vi "Set_Calibration_Settings.vi"(8 "Status/Errors in":refnum<vi>, 9 "Control Parameters [] in":T1[](array[typedef]) {"Aux Byte Value" format="%02x"; "Max Real Value" format="%#_6e"; "Min Real Value" format="%#_6e"; "dReal/dByte" format="%#_6e"; "Byte Value" format="%02x"; "Identifier" format="%02x"}, 10 "Main parameters in":T3={"Mode"={"Mode"=enum."Dialog", "Expert?"=FALSE, "Dialog?"=FALSE}, "Stop loop"={"Settings changed?"=FALSE, "Stop?"=refnum}, "Send message"={"Send mode"=enum."Get parameters", "Set parameter list"=0, "Get parameter list"=0, "Reset device"=0, "Length set settings message"=0, "Reset buttons?"=FALSE, "Reset Master?"=enum."General"}, "Write settings"={"Options"=enum."File 1"}, "Settings state"={"MAS locked?"=refnum, "SLV locked?"=refnum}, "Button refs"={"Stop program"=refnum, "Save settings"=refnum, "DAQ mode"=refnum, "Reset settings"=refnum, "Apply settings"=refnum, "Reset MAS"=refnum, "Reset SLV"=refnum, "Local DBase?"=refnum, "Last value DBase"=FALSE, "Database"=refnum, "Calibration"=refnum, "Save settings 2"=refnum}, "Update screen"={"Detector number"=0, "Hardware"=enum."None"}, "Files"={"Path config file"=path "", "Path def. ini file"=path "", "Path ini file 1"=path "", "Path ini file 2"=path "", "Path RBF file"=path ""}, "DB connection"={"connection reference"=refnum, "Connected?"=refnum, "ODBC Name"=""}, "Status_id"=refnum, "Time difference"=refnum, "Satellites"=refnum, "Alignment parameters"=refnum, "Page Statistics 2"=refnum, "Database"=refnum, "Page Statistics"=refnum} {"Update screen"."Detector number" format="%#.0f"; "Send message"."Reset device" format="%x"; "Send message"."Get parameter list" format="%x"; "Send message"."Set parameter list" format="%x"}) -> (0 "Status/Errors out":refnum<vi>, 1 "Control Parameters [] out":T1[](array[typedef]) {"Aux Byte Value" format="%02x"; "Max Real Value" format="%#_6e"; "Min Real Value" format="%#_6e"; "dReal/dByte" format="%#_6e"; "Byte Value" format="%02x"; "Identifier" format="%02x"}, 2 "Main parameters out":T3={"Mode"={"Mode"=enum."Dialog", "Expert?"=FALSE, "Dialog?"=FALSE}, "Stop loop"={"Settings changed?"=FALSE, "Stop?"=refnum}, "Send message"={"Send mode"=enum."Get parameters", "Set parameter list"=0, "Get parameter list"=0, "Reset device"=0, "Length set settings message"=0, "Reset buttons?"=FALSE, "Reset Master?"=enum."General"}, "Write settings"={"Options"=enum."File 1"}, "Settings state"={"MAS locked?"=refnum, "SLV locked?"=refnum}, "Button refs"={"Stop program"=refnum, "Save settings"=refnum, "DAQ mode"=refnum, "Reset settings"=refnum, "Apply settings"=refnum, "Reset MAS"=refnum, "Reset SLV"=refnum, "Local DBase?"=refnum, "Last value DBase"=FALSE, "Database"=refnum, "Calibration"=refnum, "Save settings 2"=refnum}, "Update screen"={"Detector number"=0, "Hardware"=enum."None"}, "Files"={"Path config file"=path "", "Path def. ini file"=path "", "Path ini file 1"=path "", "Path ini file 2"=path "", "Path RBF file"=path ""}, "DB connection"={"connection reference"=refnum, "Connected?"=refnum, "ODBC Name"=""}, "Status_id"=refnum, "Time difference"=refnum, "Satellites"=refnum, "Alignment parameters"=refnum, "Page Statistics 2"=refnum, "Database"=refnum, "Page Statistics"=refnum} {"Update screen"."Detector number" format="%#.0f"; "Send message"."Reset device" format="%x"; "Send message"."Get parameter list" format="%x"; "Send message"."Set parameter list" format="%x"})   [LabVIEW 2010]
uses:
  Controls/Main_Parameters.ctl
  Controls/Mode.ctl
  Controls/Stop_Loop.ctl
  Controls/Send_Message.ctl
  Controls/Send_Message_Mode.ctl
  Controls/Master.ctl
  Controls/Write_Settings.ctl
  Controls/Write_Settings_Options.ctl
  Controls/Settings_State.ctl
  Controls/Button_Refs.ctl
  Controls/Update_Screen.ctl
  Controls/Files.ctl
  Controls/DB_Connection.ctl
  database/Connection.llb/Conn ObjectReference.ctl
  Controls/Control_Parameters.ctl
  Controls/Get_Set_Calibration_Options.ctl
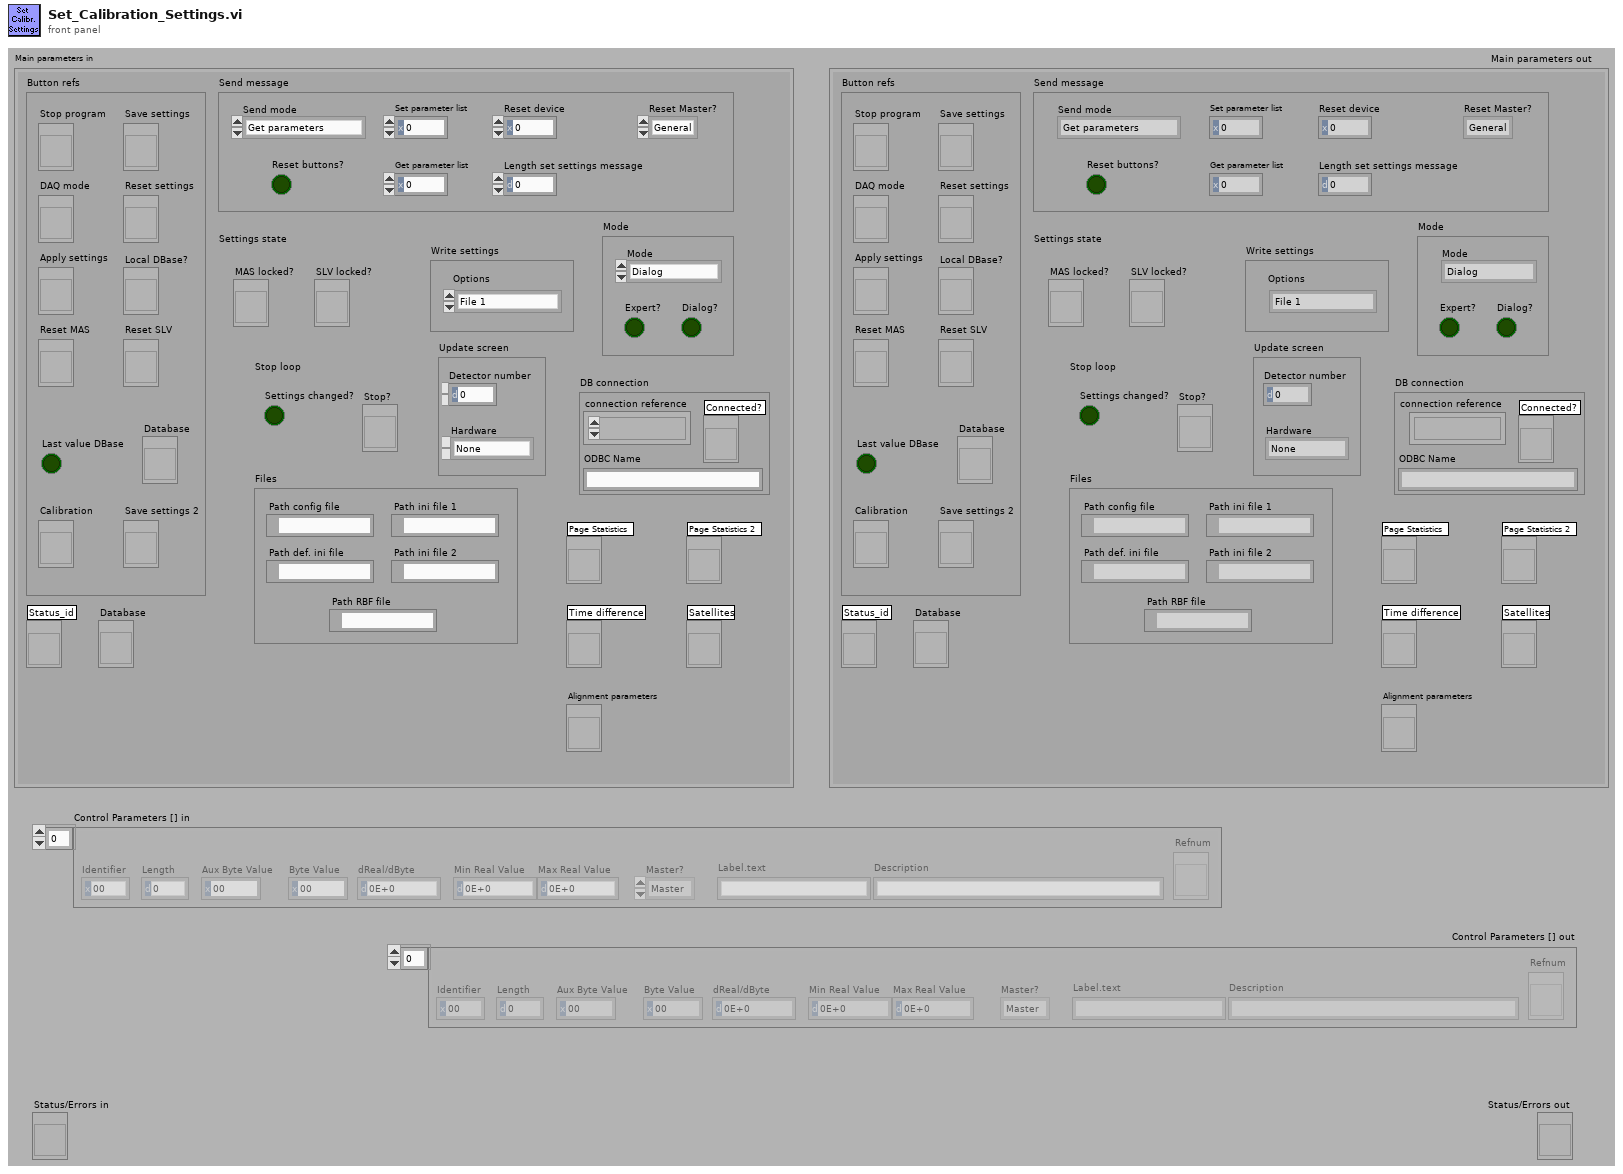
[diagram p1: front panel]
types:
  T1 = typedef "Control_Parameters.ctl" = cluster{"Identifier":u8, "Length":u16, "Byte Value":u32, "dReal/dByte":dbl, "Min Real Value":dbl, "Max Real Value":dbl, "Master?":T2, "Label.text":string, "Description":string, "Refnum":refnum<vi>, "Aux Byte Value":u32}
  T2 = typedef "Master.ctl" = enum16{"Master", "Slave", "General"}
  T3 = typedef "Main_Parameters.ctl" = cluster{"Mode":T4, "Stop loop":T5, "Send message":T6, "Write settings":T8, "Settings state":T10, "Button refs":T11, "Update screen":T12, "Files":T13, "DB connection":T14, "Status_id":refnum<vi>, "Time difference":refnum<vi>, "Satellites":refnum<vi>, "Alignment parameters":refnum<vi>, "Page Statistics 2":refnum<vi>, "Database":refnum<vi>, "Page Statistics":refnum<vi>}
  T4 = typedef "Mode.ctl" = cluster{"Mode":enum8{"Stop", "Dialog", "Hisparc II", "Hisparc II DAQ", "Alignment"}, "Expert?":bool, "Dialog?":bool}
  T5 = typedef "Stop_Loop.ctl" = cluster{"Settings changed?":bool, "Stop?":refnum<vi>}
  T6 = typedef "Send_Message.ctl" = cluster{"Send mode":T7, "Set parameter list":u8, "Get parameter list":u8, "Reset device":u8, "Length set settings message":i32, "Reset buttons?":bool, "Reset Master?":T2}
  T7 = typedef "Send_Message_Mode.ctl" = enum16{"Get parameters", "Set parameters", "From front panel", "From parameters", "Reset device", "Alignment"}
  T8 = typedef "Write_Settings.ctl" = cluster{"Options":T9}
  T9 = typedef "Write_Settings_Options.ctl" = enum16{"File 1", "File 2", "Alignment", "Reset"}
  T10 = typedef "Settings_State.ctl" = cluster{"MAS locked?":refnum<vi>, "SLV locked?":refnum<vi>}
  T11 = typedef "Button_Refs.ctl" = cluster{"Stop program":refnum<vi>, "Save settings":refnum<vi>, "DAQ mode":refnum<vi>, "Reset settings":refnum<vi>, "Apply settings":refnum<vi>, "Reset MAS":refnum<vi>, "Reset SLV":refnum<vi>, "Local DBase?":refnum<vi>, "Last value DBase":bool, "Database":refnum<vi>, "Calibration":refnum<vi>, "Save settings 2":refnum<vi>}
  T12 = typedef "Update_Screen.ctl" = cluster{"Detector number":u16, "Hardware":enum8{"None", "HiSPARC I", "HiSPARC II", "HiSPARC III", "Unknown"}}
  T13 = typedef "Files.ctl" = cluster{"Path config file":path, "Path def. ini file":path, "Path ini file 1":path, "Path ini file 2":path, "Path RBF file":path}
  T14 = typedef "DB_Connection.ctl" = cluster{"connection reference":T15, "Connected?":refnum<vi>, "ODBC Name":string}
  T15 = typedef "Conn ObjectReference.ctl" = refnum<k1>
  T16 = typedef "Get_Set_Calibration_Options.ctl" = enum16{"Get", "Set", "Set MAS", "Set SLV"}
  T17 = typedef "Calibration_Parameters.ctl" = cluster{"New settings MAS?":bool, "New settings SLV?":bool, "Alignment step MAS":i32, "Alignment step SLV":i32, "MAS Ch. 1":cluster{"Offset adjust pos.":u8, "Offset adjust neg.":u8, "Gain adjust pos.":u8, "Gain adjust neg.":u8, "Count pos.":dbl, "Count neg.":dbl}, "MAS Ch. 2":cluster{"Offset adjust pos.":u8, "Offset adjust neg.":u8, "Gain adjust pos.":u8, "Gain adjust neg.":u8, "Count pos.":dbl, "Count neg.":dbl}, "SLV Ch. 1":cluster{"Offset adjust pos.":u8, "Offset adjust neg.":u8, "Gain adjust pos.":u8, "Gain adjust neg.":u8, "Count pos.":dbl, "Count neg.":dbl}, "SLV Ch. 2":cluster{"Offset adjust pos.":u8, "Offset adjust neg.":u8, "Gain adjust pos.":u8, "Gain adjust neg.":u8, "Count pos.":dbl, "Count neg.":dbl}, "Comm. offset MAS":u8, "Full scale MAS":u8, "Comm. offset SLV":u8, "Full scale SLV":u8, "Trigger condition":u8, "Pre coinc. time":u16, "Coinc. time":u16, "Post coinc. time":u16, "Hardware":enum8{"None", "HiSPARC I", "HiSPARC II", "HiSPARC III", "Unknown"}}
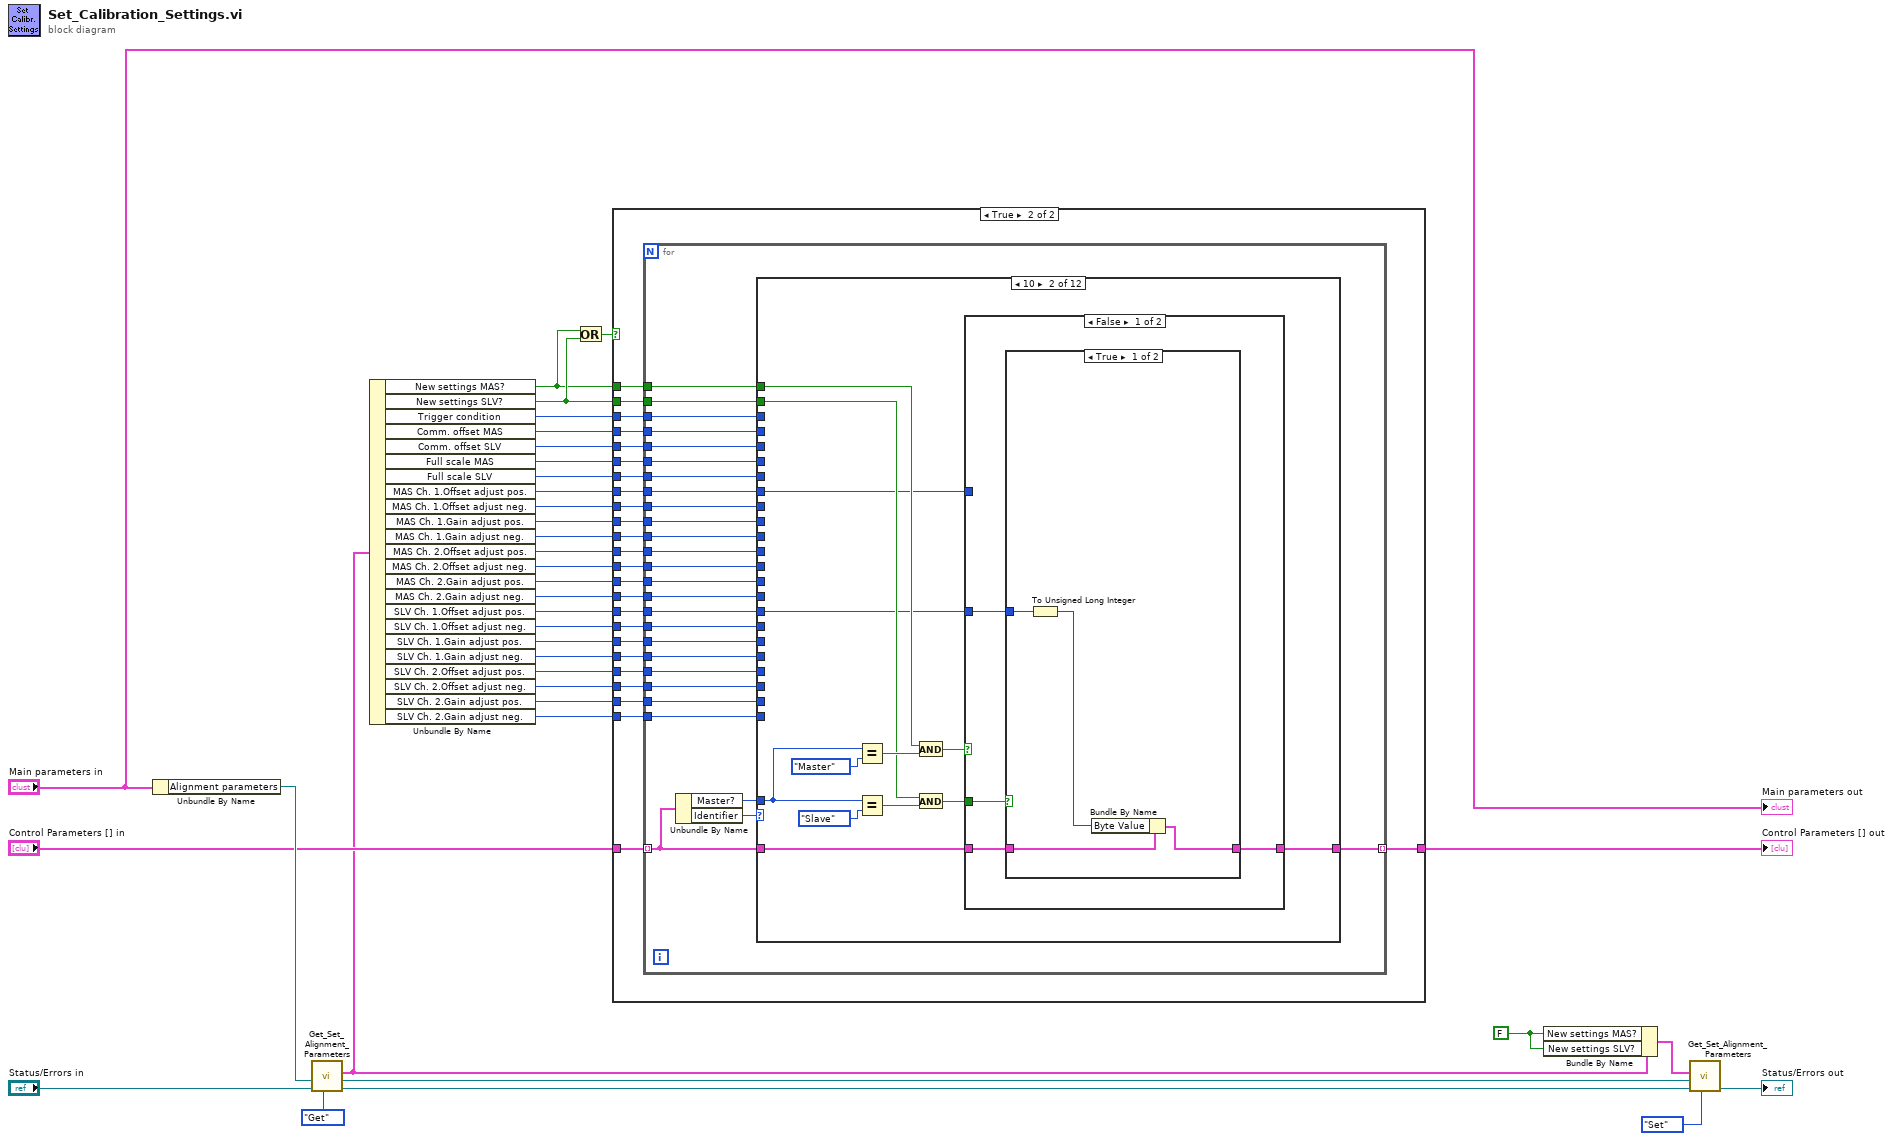
[diagram p0: block diagram]
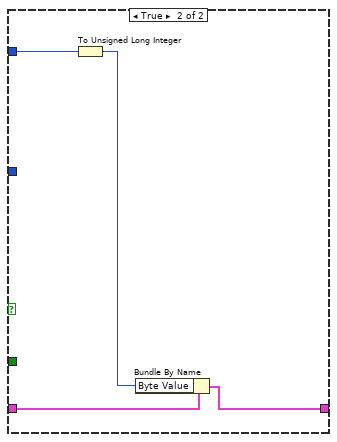
[diagram p5: hidden frame]
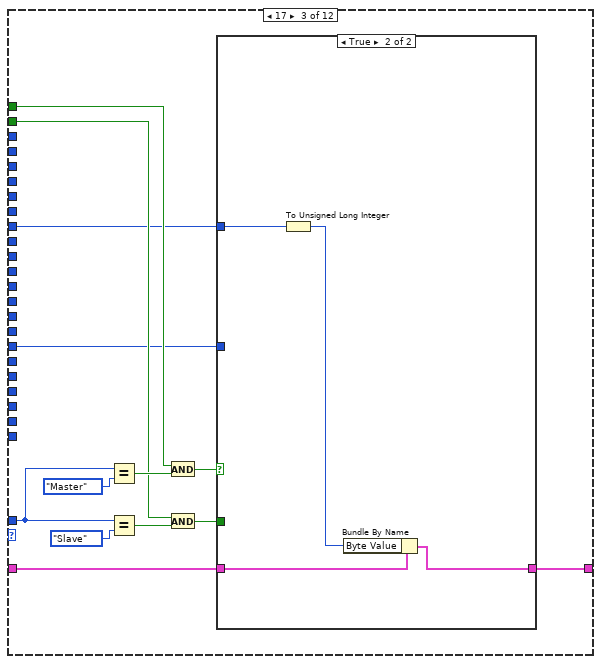
[diagram p6: hidden frame]
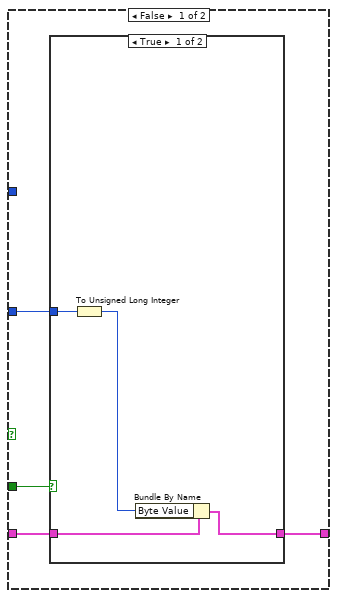
[diagram p7: hidden frame]
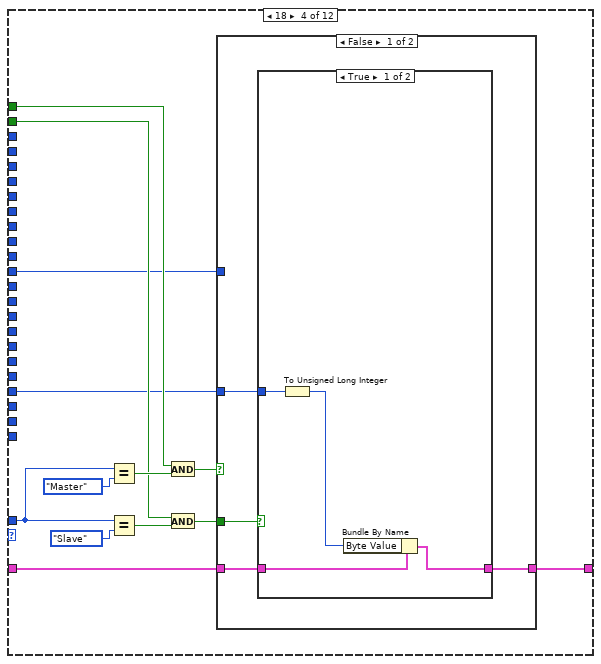
[diagram p9: hidden frame]
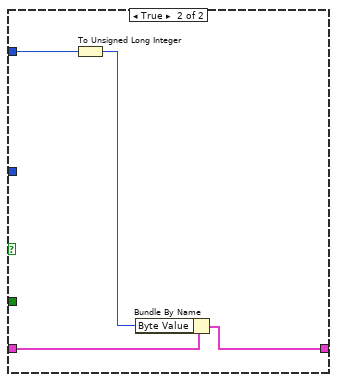
[diagram p11: hidden frame]
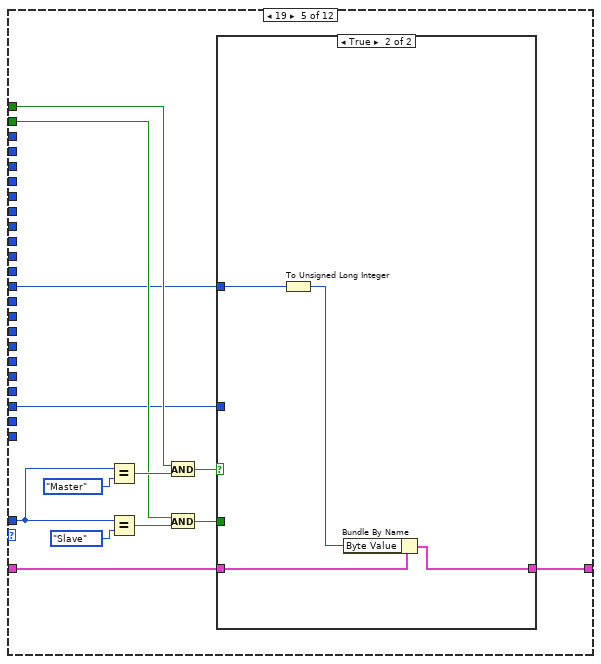
[diagram p12: hidden frame]
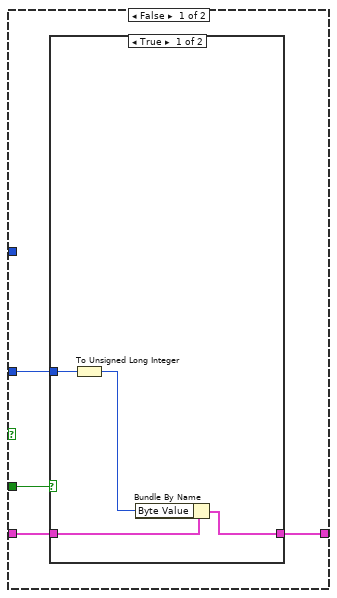
[diagram p13: hidden frame]
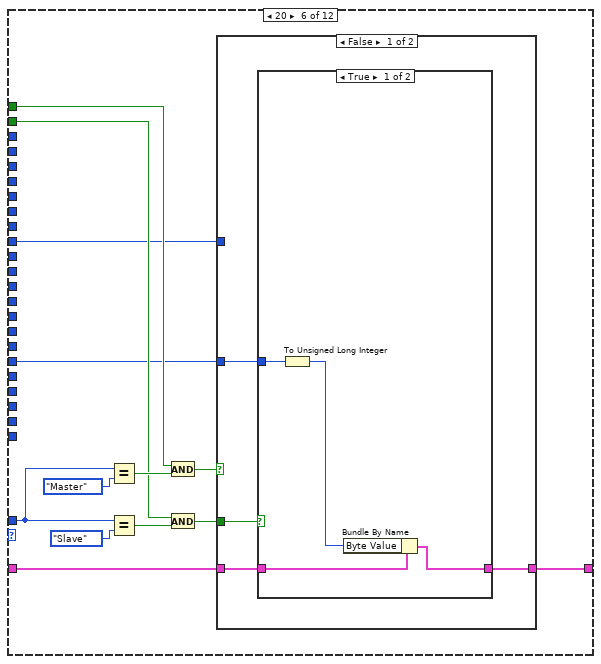
[diagram p15: hidden frame]
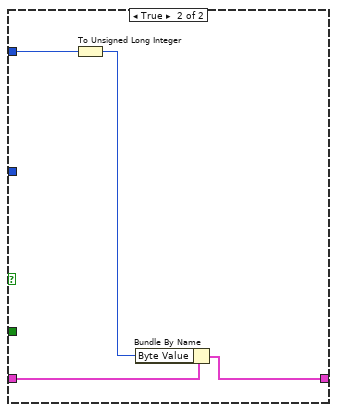
[diagram p17: hidden frame]
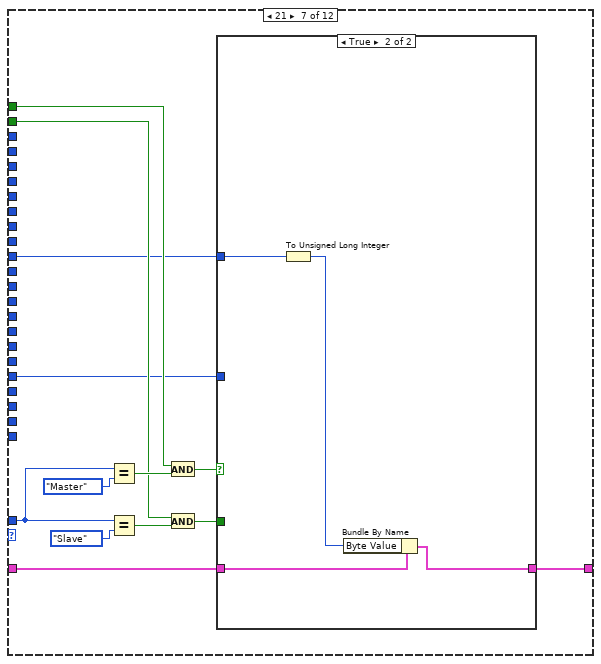
[diagram p18: hidden frame]
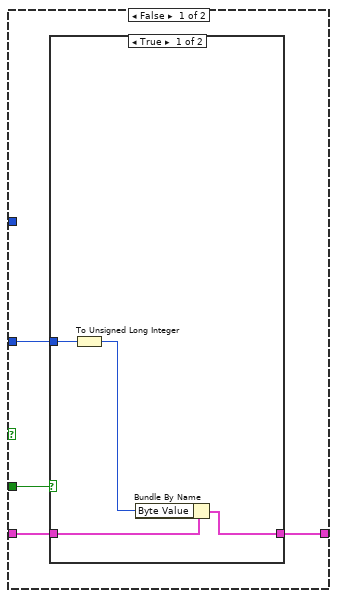
[diagram p19: hidden frame]
diagram:
  w6 = FALSE ("New settings MAS?")
  n1 = Unbundle By Name("Main parameters in") -> ("Alignment parameters"=w35:refnum<vi>)
  n2 = call "Get_Set_Alignment_Parameters.vi"("Get/Set"=Get_Set_Calibration_Options."Get", "Status/Errors in"="Status/Errors in", "Alignment parameters in"=w35) -> ("Status/Errors out"=w11:refnum<vi>, "Alignment parameters out"=w7:refnum<vi>, "Value out"=w9:T17)  [unwired: 2 in, 4 out]
  n3 = Unbundle By Name(w9) -> ("New settings MAS?"=w3:bool, "New settings SLV?"=w4:bool, "Trigger condition"=w31:u8, "Comm. offset MAS"=w30:u8, "Comm. offset SLV"=w2:u8, "Full scale MAS"=w29:u8, "Full scale SLV"=w1:u8, "MAS Ch. 1.Offset adjust pos."=w28:u8, "MAS Ch. 1.Offset adjust neg."=w27:u8, "MAS Ch. 1.Gain adjust pos."=w26:u8, "MAS Ch. 1.Gain adjust neg."=w25:u8, "MAS Ch. 2.Offset adjust pos."=w24:u8, "MAS Ch. 2.Offset adjust neg."=w23:u8, "MAS Ch. 2.Gain adjust pos."=w22:u8, "MAS Ch. 2.Gain adjust neg."=w21:u8, "SLV Ch. 1.Offset adjust pos."=w20:u8, "SLV Ch. 1.Offset adjust neg."=w19:u8, "SLV Ch. 1.Gain adjust pos."=w18:u8, "SLV Ch. 1.Gain adjust neg."=w17:u8, "SLV Ch. 2.Offset adjust pos."=w16:u8, "SLV Ch. 2.Offset adjust neg."=w15:u8, "SLV Ch. 2.Gain adjust pos."=w14:u8, "SLV Ch. 2.Gain adjust neg."=w13:u8)
  n4 = Or(x=w3, y=w4) -> (x .or. y?=w5:bool)
  n5 = case shown="True" w5 {
    tunnel: "Control Parameters [] in" -> [w38 w63]
    tunnel: w3 -> [_ w62]
    tunnel: w4 -> [_ w61]
    tunnel: [w38 w60] -> w33
    tunnel: w31 -> [_ w59]
    tunnel: w30 -> [_ w58]
    tunnel: w29 -> [_ w57]
    tunnel: w28 -> [_ w56]
    tunnel: w27 -> [_ w55]
    tunnel: w26 -> [_ w54]
    tunnel: w25 -> [_ w53]
    tunnel: w24 -> [_ w52]
    tunnel: w23 -> [_ w51]
    tunnel: w22 -> [_ w50]
    tunnel: w21 -> [_ w49]
    tunnel: w20 -> [_ w48]
    tunnel: w19 -> [_ w47]
    tunnel: w18 -> [_ w46]
    tunnel: w17 -> [_ w45]
    tunnel: w16 -> [_ w44]
    tunnel: w15 -> [_ w43]
    tunnel: w14 -> [_ w42]
    tunnel: w13 -> [_ w41]
    tunnel: w2 -> [_ w40]
    tunnel: w1 -> [_ w39]
    frame False {
    }
    frame True {
      n6 = for {
        tunnel: w63 -> [w67] mode=indexing
        tunnel: w62 -> [w89]
        tunnel: w61 -> [w88]
        tunnel: [w68] -> w60 mode=indexing
        tunnel: w59 -> [w87]
        tunnel: w58 -> [w86]
        tunnel: w57 -> [w85]
        tunnel: w56 -> [w84]
        tunnel: w55 -> [w83]
        tunnel: w54 -> [w82]
        tunnel: w53 -> [w81]
        tunnel: w52 -> [w80]
        tunnel: w51 -> [w79]
        tunnel: w50 -> [w78]
        tunnel: w49 -> [w77]
        tunnel: w48 -> [w76]
        tunnel: w47 -> [w75]
        tunnel: w46 -> [w74]
        tunnel: w45 -> [w73]
        tunnel: w44 -> [w72]
        tunnel: w43 -> [w71]
        tunnel: w42 -> [w70]
        tunnel: w41 -> [w69]
        tunnel: w40 -> [w65]
        tunnel: w39 -> [w64]
        n7 = Unbundle By Name(w67) -> ("Master?"=w66:T2, "Identifier"=w90:u8)
        n8 = case shown="10" w90 {
          tunnel: w89 -> [_ w97 w123 w149 w175 w201 w227 w253 w279 w305 w331 _]
          tunnel: w88 -> [_ w96 w122 w148 w174 w200 w226 w252 w278 w304 w330 _]
          tunnel: w87 -> [_ _ _ _ _ _ _ _ _ _ _ w352]
          tunnel: w86 -> [_ _ _ _ _ _ _ _ _ w300 _ _]
          tunnel: w85 -> [_ _ _ _ _ _ _ _ _ _ w327 _]
          tunnel: w84 -> [_ w93 _ _ _ _ _ _ _ _ _ _]
          tunnel: w83 -> [_ _ w119 _ _ _ _ _ _ _ _ _]
          tunnel: w82 -> [_ _ _ _ _ w197 _ _ _ _ _ _]
          tunnel: w81 -> [_ _ _ _ _ _ w223 _ _ _ _ _]
          tunnel: w80 -> [_ _ _ w145 _ _ _ _ _ _ _ _]
          tunnel: w79 -> [_ _ _ _ w171 _ _ _ _ _ _ _]
          tunnel: w78 -> [_ _ _ _ _ _ _ w249 _ _ _ _]
          tunnel: w77 -> [_ _ _ _ _ _ _ _ w275 _ _ _]
          tunnel: w76 -> [_ w92 _ _ _ _ _ _ _ _ _ _]
          tunnel: w75 -> [_ _ w118 _ _ _ _ _ _ _ _ _]
          tunnel: w74 -> [_ _ _ _ _ w196 _ _ _ _ _ _]
          tunnel: w73 -> [_ _ _ _ _ _ w222 _ _ _ _ _]
          tunnel: w72 -> [_ _ _ w144 _ _ _ _ _ _ _ _]
          tunnel: w71 -> [_ _ _ _ w170 _ _ _ _ _ _ _]
          tunnel: w70 -> [_ _ _ _ _ _ _ w248 _ _ _ _]
          tunnel: w69 -> [_ _ _ _ _ _ _ _ w274 _ _ _]
          tunnel: [w91 w104 w130 w156 w182 w208 w234 w260 w286 w312 w338 w353] -> w68
          tunnel: w67 -> [w91 w103 w129 w155 w181 w207 w233 w259 w285 w311 w337 w354]
          tunnel: w66 -> [_ w98 w124 w150 w176 w202 w228 w254 w280 w306 w332 _]
          tunnel: w65 -> [_ _ _ _ _ _ _ _ _ w301 _ _]
          tunnel: w64 -> [_ _ _ _ _ _ _ _ _ _ w326 _]
          frame Default {
          }
          frame 16 {
            n9 = Equal?(x=w98, y=Master."Master") -> (x = y?=w99:bool)
            n10 = Equal?(x=w98, y=Master."Slave") -> (x = y?=w101:bool)
            n11 = And(x=w97, y=w99) -> (x .and. y?=w95:bool)
            n12 = And(x=w96, y=w101) -> (x .and. y?=w94:bool)
            n13 = case shown="False" w95 {
              tunnel: [w108 w115] -> w104
              tunnel: w103 -> [w107 w116]
              tunnel: w94 -> [w106 _]
              tunnel: w93 -> [_ w114]
              tunnel: w92 -> [w105 _]
              frame False {
                n14 = case shown="True" w106 {
                  tunnel: [w112 w113] -> w108
                  tunnel: w107 -> [w111 w113]
                  tunnel: w105 -> [w110 _]
                  frame True {
                    n15 = To Unsigned Long Integer(number=w110) -> (unsigned 32bit integer=w109:u32)
                    n16 = Bundle By Name(cluster=w111, "Byte Value"=w109) -> (w112:T1)
                  }
                  frame False, Default {
                  }
                }
              }
              frame True {
                n17 = To Unsigned Long Integer(number=w114) -> (unsigned 32bit integer=w117:u32)
                n18 = Bundle By Name(cluster=w116, "Byte Value"=w117) -> (w115:T1)
              }
            }
          }
          frame 17 {
            n19 = Equal?(x=w124, y=Master."Master") -> (x = y?=w125:bool)
            n20 = Equal?(x=w124, y=Master."Slave") -> (x = y?=w127:bool)
            n21 = And(x=w123, y=w125) -> (x .and. y?=w121:bool)
            n22 = And(x=w122, y=w127) -> (x .and. y?=w120:bool)
            n23 = case shown="True" w121 {
              tunnel: [w134 w141] -> w130
              tunnel: w129 -> [w133 w142]
              tunnel: w120 -> [w132 _]
              tunnel: w118 -> [w131 _]
              tunnel: w119 -> [_ w140]
              frame False {
                n24 = case shown="True" w132 {
                  tunnel: [w138 w139] -> w134
                  tunnel: w133 -> [w137 w139]
                  tunnel: w131 -> [w136 _]
                  frame True {
                    n25 = To Unsigned Long Integer(number=w136) -> (unsigned 32bit integer=w135:u32)
                    n26 = Bundle By Name(cluster=w137, "Byte Value"=w135) -> (w138:T1)
                  }
                  frame False, Default {
                  }
                }
              }
              frame True {
                n27 = To Unsigned Long Integer(number=w140) -> (unsigned 32bit integer=w143:u32)
                n28 = Bundle By Name(cluster=w142, "Byte Value"=w143) -> (w141:T1)
              }
            }
          }
          frame 18 {
            n29 = Equal?(x=w150, y=Master."Master") -> (x = y?=w151:bool)
            n30 = Equal?(x=w150, y=Master."Slave") -> (x = y?=w153:bool)
            n31 = And(x=w149, y=w151) -> (x .and. y?=w147:bool)
            n32 = And(x=w148, y=w153) -> (x .and. y?=w146:bool)
            n33 = case shown="False" w147 {
              tunnel: [w160 w167] -> w156
              tunnel: w155 -> [w159 w168]
              tunnel: w146 -> [w158 _]
              tunnel: w144 -> [w157 _]
              tunnel: w145 -> [_ w166]
              frame False {
                n34 = case shown="True" w158 {
                  tunnel: [w164 w165] -> w160
                  tunnel: w159 -> [w163 w165]
                  tunnel: w157 -> [w162 _]
                  frame True {
                    n35 = To Unsigned Long Integer(number=w162) -> (unsigned 32bit integer=w161:u32)
                    n36 = Bundle By Name(cluster=w163, "Byte Value"=w161) -> (w164:T1)
                  }
                  frame False, Default {
                  }
                }
              }
              frame True {
                n37 = To Unsigned Long Integer(number=w166) -> (unsigned 32bit integer=w169:u32)
                n38 = Bundle By Name(cluster=w168, "Byte Value"=w169) -> (w167:T1)
              }
            }
          }
          frame 19 {
            n39 = Equal?(x=w176, y=Master."Master") -> (x = y?=w177:bool)
            n40 = Equal?(x=w176, y=Master."Slave") -> (x = y?=w179:bool)
            n41 = And(x=w175, y=w177) -> (x .and. y?=w173:bool)
            n42 = And(x=w174, y=w179) -> (x .and. y?=w172:bool)
            n43 = case shown="True" w173 {
              tunnel: [w186 w193] -> w182
              tunnel: w181 -> [w185 w194]
              tunnel: w172 -> [w184 _]
              tunnel: w170 -> [w183 _]
              tunnel: w171 -> [_ w192]
              frame False {
                n44 = case shown="True" w184 {
                  tunnel: [w190 w191] -> w186
                  tunnel: w185 -> [w189 w191]
                  tunnel: w183 -> [w188 _]
                  frame True {
                    n45 = To Unsigned Long Integer(number=w188) -> (unsigned 32bit integer=w187:u32)
                    n46 = Bundle By Name(cluster=w189, "Byte Value"=w187) -> (w190:T1)
                  }
                  frame False, Default {
                  }
                }
              }
              frame True {
                n47 = To Unsigned Long Integer(number=w192) -> (unsigned 32bit integer=w195:u32)
                n48 = Bundle By Name(cluster=w194, "Byte Value"=w195) -> (w193:T1)
              }
            }
          }
          frame 20 {
            n49 = Equal?(x=w202, y=Master."Master") -> (x = y?=w203:bool)
            n50 = Equal?(x=w202, y=Master."Slave") -> (x = y?=w205:bool)
            n51 = And(x=w201, y=w203) -> (x .and. y?=w199:bool)
            n52 = And(x=w200, y=w205) -> (x .and. y?=w198:bool)
            n53 = case shown="False" w199 {
              tunnel: [w212 w219] -> w208
              tunnel: w207 -> [w211 w220]
              tunnel: w198 -> [w210 _]
              tunnel: w196 -> [w209 _]
              tunnel: w197 -> [_ w218]
              frame False {
                n54 = case shown="True" w210 {
                  tunnel: [w216 w217] -> w212
                  tunnel: w211 -> [w215 w217]
                  tunnel: w209 -> [w214 _]
                  frame True {
                    n55 = To Unsigned Long Integer(number=w214) -> (unsigned 32bit integer=w213:u32)
                    n56 = Bundle By Name(cluster=w215, "Byte Value"=w213) -> (w216:T1)
                  }
                  frame False, Default {
                  }
                }
              }
              frame True {
                n57 = To Unsigned Long Integer(number=w218) -> (unsigned 32bit integer=w221:u32)
                n58 = Bundle By Name(cluster=w220, "Byte Value"=w221) -> (w219:T1)
              }
            }
          }
          frame 21 {
            n59 = Equal?(x=w228, y=Master."Master") -> (x = y?=w229:bool)
            n60 = Equal?(x=w228, y=Master."Slave") -> (x = y?=w231:bool)
            n61 = And(x=w227, y=w229) -> (x .and. y?=w225:bool)
            n62 = And(x=w226, y=w231) -> (x .and. y?=w224:bool)
            n63 = case shown="True" w225 {
              tunnel: [w238 w245] -> w234
              tunnel: w233 -> [w237 w246]
              tunnel: w224 -> [w236 _]
              tunnel: w222 -> [w235 _]
              tunnel: w223 -> [_ w244]
              frame False {
                n64 = case shown="True" w236 {
                  tunnel: [w242 w243] -> w238
                  tunnel: w237 -> [w241 w243]
                  tunnel: w235 -> [w240 _]
                  frame True {
                    n65 = To Unsigned Long Integer(number=w240) -> (unsigned 32bit integer=w239:u32)
                    n66 = Bundle By Name(cluster=w241, "Byte Value"=w239) -> (w242:T1)
                  }
                  frame False, Default {
                  }
                }
              }
              frame True {
                n67 = To Unsigned Long Integer(number=w244) -> (unsigned 32bit integer=w247:u32)
                n68 = Bundle By Name(cluster=w246, "Byte Value"=w247) -> (w245:T1)
              }
            }
          }
          frame 22 {
            n69 = Equal?(x=w254, y=Master."Master") -> (x = y?=w255:bool)
            n70 = Equal?(x=w254, y=Master."Slave") -> (x = y?=w257:bool)
            n71 = And(x=w253, y=w255) -> (x .and. y?=w251:bool)
            n72 = And(x=w252, y=w257) -> (x .and. y?=w250:bool)
            n73 = case shown="False" w251 {
              tunnel: [w264 w271] -> w260
              tunnel: w259 -> [w263 w272]
              tunnel: w250 -> [w262 _]
              tunnel: w248 -> [w261 _]
              tunnel: w249 -> [_ w270]
              frame False {
                n74 = case shown="True" w262 {
                  tunnel: [w268 w269] -> w264
                  tunnel: w263 -> [w267 w269]
                  tunnel: w261 -> [w266 _]
                  frame True {
                    n75 = To Unsigned Long Integer(number=w266) -> (unsigned 32bit integer=w265:u32)
                    n76 = Bundle By Name(cluster=w267, "Byte Value"=w265) -> (w268:T1)
                  }
                  frame False, Default {
                  }
                }
              }
              frame True {
                n77 = To Unsigned Long Integer(number=w270) -> (unsigned 32bit integer=w273:u32)
                n78 = Bundle By Name(cluster=w272, "Byte Value"=w273) -> (w271:T1)
              }
            }
          }
          frame 23 {
            n79 = Equal?(x=w280, y=Master."Master") -> (x = y?=w281:bool)
            n80 = Equal?(x=w280, y=Master."Slave") -> (x = y?=w283:bool)
            n81 = And(x=w279, y=w281) -> (x .and. y?=w277:bool)
            n82 = And(x=w278, y=w283) -> (x .and. y?=w276:bool)
            n83 = case shown="True" w277 {
              tunnel: [w290 w297] -> w286
              tunnel: w285 -> [w289 w298]
              tunnel: w276 -> [w288 _]
              tunnel: w274 -> [w287 _]
              tunnel: w275 -> [_ w296]
              frame False {
                n84 = case shown="True" w288 {
                  tunnel: [w294 w295] -> w290
                  tunnel: w289 -> [w293 w295]
                  tunnel: w287 -> [w292 _]
                  frame True {
                    n85 = To Unsigned Long Integer(number=w292) -> (unsigned 32bit integer=w291:u32)
                    n86 = Bundle By Name(cluster=w293, "Byte Value"=w291) -> (w294:T1)
                  }
                  frame False, Default {
                  }
                }
              }
              frame True {
                n87 = To Unsigned Long Integer(number=w296) -> (unsigned 32bit integer=w299:u32)
                n88 = Bundle By Name(cluster=w298, "Byte Value"=w299) -> (w297:T1)
              }
            }
          }
          frame 24 {
            n89 = Equal?(x=w306, y=Master."Master") -> (x = y?=w307:bool)
            n90 = Equal?(x=w306, y=Master."Slave") -> (x = y?=w309:bool)
            n91 = And(x=w305, y=w307) -> (x .and. y?=w303:bool)
            n92 = And(x=w304, y=w309) -> (x .and. y?=w302:bool)
            n93 = case shown="True" w303 {
              tunnel: [w316 w323] -> w312
              tunnel: w311 -> [w315 w324]
              tunnel: w302 -> [w314 _]
              tunnel: w301 -> [w313 _]
              tunnel: w300 -> [_ w322]
              frame False {
                n94 = case shown="True" w314 {
                  tunnel: [w320 w321] -> w316
                  tunnel: w315 -> [w319 w321]
                  tunnel: w313 -> [w318 _]
                  frame True {
                    n95 = To Unsigned Long Integer(number=w318) -> (unsigned 32bit integer=w317:u32)
                    n96 = Bundle By Name(cluster=w319, "Byte Value"=w317) -> (w320:T1)
                  }
                  frame False, Default {
                  }
                }
              }
              frame True {
                n97 = To Unsigned Long Integer(number=w322) -> (unsigned 32bit integer=w325:u32)
                n98 = Bundle By Name(cluster=w324, "Byte Value"=w325) -> (w323:T1)
              }
            }
          }
          frame 25 {
            n99 = Equal?(x=w332, y=Master."Master") -> (x = y?=w333:bool)
            n100 = Equal?(x=w332, y=Master."Slave") -> (x = y?=w335:bool)
            n101 = And(x=w331, y=w333) -> (x .and. y?=w329:bool)
            n102 = And(x=w330, y=w335) -> (x .and. y?=w328:bool)
            n103 = case shown="False" w329 {
              tunnel: [w342 w349] -> w338
              tunnel: w337 -> [w341 w350]
              tunnel: w328 -> [w340 _]
              tunnel: w327 -> [_ w348]
              tunnel: w326 -> [w339 _]
              frame False {
                n104 = case shown="True" w340 {
                  tunnel: [w346 w347] -> w342
                  tunnel: w341 -> [w345 w347]
                  tunnel: w339 -> [w344 _]
                  frame True {
                    n105 = To Unsigned Long Integer(number=w344) -> (unsigned 32bit integer=w343:u32)
                    n106 = Bundle By Name(cluster=w345, "Byte Value"=w343) -> (w346:T1)
                  }
                  frame False, Default {
                  }
                }
              }
              frame True {
                n107 = To Unsigned Long Integer(number=w348) -> (unsigned 32bit integer=w351:u32)
                n108 = Bundle By Name(cluster=w350, "Byte Value"=w351) -> (w349:T1)
              }
            }
          }
          frame 48 {
            n109 = To Unsigned Long Integer(number=w352) -> (unsigned 32bit integer=w355:u32)
            n110 = Bundle By Name(cluster=w354, "Byte Value"=w355) -> (w353:T1)
          }
        }
      }
    }
  }
  "Control Parameters [] out" <- w33
  n111 = Bundle By Name(cluster=w9, "New settings MAS?"=w6, "New settings SLV?"=w6) -> (w8:T17)
  n112 = call "Get_Set_Alignment_Parameters.vi"("Get/Set"=Get_Set_Calibration_Options."Set", "Status/Errors in"=w11, "Alignment parameters in"=w7, "Value in"=w8) -> ("Status/Errors out"=→"Status/Errors out":refnum<vi>)  [unwired: 1 in, 6 out]
  "Main parameters out" <- "Main parameters in"
